vi "Normalized Range Compare 2016.vi"(2 "Y Averages":dbl[](graph), 3 "X Averages":dbl[](graph)) -> (0 "Y Score":dbl, 1 "X Score":dbl)   [LabVIEW 2016]
doc: "The input data represents the average pixels set for each row and each column of the possible target. Since targets are expected to have hollow portions, covered in tape, compare the pixels average to the expected min and max values across the target. Higher scores indicate the averages fit the expected profiles."
panel:
  out "Y Results":dbl[][](graph)
  in  "Y Min":dbl[](array[numeric])=[0.0, 0.1, 0.1, 0.1, 0.1, 0.1, 0.1, 0.1, 0.1, 0.1, 0.1, 0.1, 0.2, 0.7, 0.0]
  in  "Y Max":dbl[](array[numeric])=[0.4, 0.4, 0.4, 0.4, 0.4, 0.4, 0.4, 0.4, 0.4, 0.4, 0.4, 1.0, 1.0, 1.0, 1.0]
  in  "X Min":dbl[](array[numeric])=[0.1, 0.7, 0.1, 0.05, 0.05, 0.05, 0.05, 0.05, 0.05, 0.05, 0.05, 0.05, 0.05, 0.05, 0.05, 0.05, 0.05, 0.05, 0.05, 0.05, 0.05, 0.1, 0.7, 0.1]
  out "X Results":dbl[][](graph)
  in  "X Max":dbl[](array[numeric])=[1.0, 1.0, 1.0, 1.0, 1.0, 0.3, 0.3, 0.3, 0.3, 0.3, 0.3, 0.3, 0.3, 0.3, 0.3, 0.3, 0.3, 0.3, 0.3, 1.0, 1.0, 1.0, 1.0, 1.0]
  # "Measure the average pixel row/column values against the limits, counting how many are between the min and max. \nThe top graphs are vertical pixel columns and looks something like the actual target.\nThe bottom graphs are still sideways and are the sum of rows."
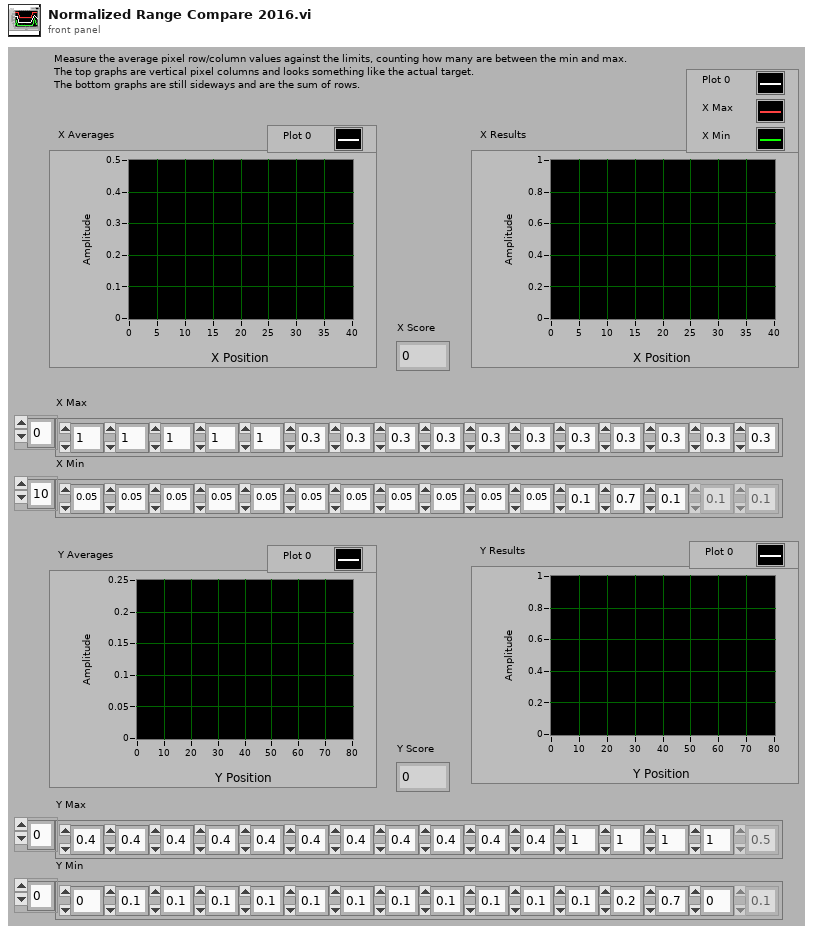
[diagram p1: front panel]
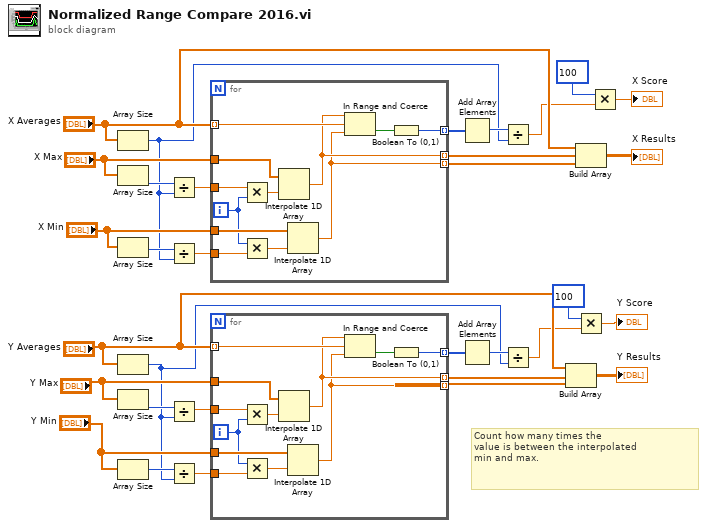
[diagram p0: block diagram]
diagram:
  # "Count how many times the\nvalue is between the interpolated\nmin and max."
  n1 = Array Size(array="X Averages") -> (size(s)=w8:i32)
  n2 = Array Size(array="X Max") -> (size(s)=w27:i32)
  n3 = Array Size(array="X Min") -> (size(s)=w16:i32)
  n4 = Array Size(array="Y Averages") -> (size(s)=w7:i32)
  n5 = Array Size(array="Y Max") -> (size(s)=w25:i32)
  n6 = Array Size(array="Y Min") -> (size(s)=w18:i32)
  n7 = Divide(x=w27, y=w8) -> (x/y=w26:dbl)
  n8 = Divide(x=w16, y=w8) -> (x/y=w14:dbl)
  n9 = Divide(x=w25, y=w7) -> (x/y=w23:dbl)
  n10 = Divide(x=w18, y=w7) -> (x/y=w13:dbl)
  n11 = for {
    tunnel: "X Averages" -> [w44] mode=indexing
    tunnel: "X Max" -> [w42]
    tunnel: [w41] -> w32 mode=indexing
    tunnel: [w38] -> w31 mode=indexing
    tunnel: w26 -> [w43]
    tunnel: "X Min" -> [w40]
    tunnel: w14 -> [w36]
    tunnel: [w33] -> w12 mode=indexing
    i -> [w37]
    n12 = Multiply(x=w43, y=w37) -> (x*y=w39:dbl)
    n13 = Multiply(x=w37, y=w36) -> (x*y=w35:dbl)
    n14 = Interpolate 1D Array(1:w39, 2:w42) -> (0:w41:dbl)
    n15 = Interpolate 1D Array(1:w35, 2:w40) -> (0:w38:dbl)
    n16 = In Range and Coerce(upper limit=w41, x=w44, lower limit=w38) -> (In Range?=w34:bool)  [unwired: 1 out]
    n17 = Boolean To (0,1)(Boolean=w34) -> (0, 1=w33:i16)
  }
  n18 = for {
    tunnel: "Y Averages" -> [w56] mode=indexing
    tunnel: "Y Max" -> [w54]
    tunnel: [w53] -> w21 mode=indexing
    tunnel: [w50] -> w20 mode=indexing
    tunnel: w23 -> [w55]
    tunnel: "Y Min" -> [w52]
    tunnel: w13 -> [w47]
    tunnel: [w45] -> w11 mode=indexing
    i -> [w49]
    n19 = Multiply(x=w55, y=w49) -> (x*y=w51:dbl)
    n20 = Multiply(x=w49, y=w47) -> (x*y=w48:dbl)
    n21 = Interpolate 1D Array(1:w51, 2:w54) -> (0:w53:dbl)
    n22 = Interpolate 1D Array(1:w48, 2:w52) -> (0:w50:dbl)
    n23 = In Range and Coerce(upper limit=w53, x=w56, lower limit=w50) -> (In Range?=w46:bool)  [unwired: 1 out]
    n24 = Boolean To (0,1)(Boolean=w46) -> (0, 1=w45:i16)
  }
  n25 = Add Array Elements(numeric array=w12) -> (sum=w9:i16)
  n26 = Add Array Elements(numeric array=w11) -> (sum=w10:i16)
  n27 = Divide(x=w9, y=w8) -> (x/y=w6:dbl)
  n28 = Divide(x=w10, y=w7) -> (x/y=w3:dbl)
  n29 = Build Array("Y Averages", w21, w20) -> (→"Y Results":dbl[][])
  n30 = Build Array("X Averages", w32, w31) -> (→"X Results":dbl[][])
  n31 = Multiply(x=100, y=w3) -> (x*y=→"Y Score":dbl)
  n32 = Multiply(x=100, y=w6) -> (x*y=→"X Score":dbl)
